vi "Benchmarking Sets.vi"() -> ()   [LabVIEW 2019]
uses:
  60997348-983d-410f-b173-2636c18fe73e.vi
  dff44dff-3936-4863-b921-07dd1a0d616c.vi
  04c840ee-3486-441b-89c1-6d55a373077b.vi
  1b5ecc8c-3254-42fc-b27c-bc730ca8b5e0.vi
  041710f1-907d-468f-a1fd-b8ae1aa895de.vi
panel:
  out "Array Intersection Count":i32
  out "Array Sym Diff Count":i32
  out "Array Union Count":i32
  out "Array Diff Count":i32
  out "Set Intersection Complete":bool=TRUE
  out "Set Intersection Started":bool=TRUE
  out "Set Symmetric Diff Complete":bool=TRUE
  out "Set Symmetric Diff Started":bool=TRUE
  out "Set Union Complete":bool=TRUE
  out "Set Union Started":bool=TRUE
  out "Set Diff Complete":bool=TRUE
  out "Set Diff Started":bool=TRUE
  out "Set Build Complete":bool=TRUE
  out "Set Build Started":bool=TRUE
  out "Array Intersection Complete":bool=TRUE
  out "Array Intersection Started":bool=TRUE
  out "Array Symmetric Diff Complete":bool=TRUE
  out "Array Symmetric Diff Started":bool=TRUE
  out "Array Union Complete":bool=TRUE
  out "Array Union Started":bool=TRUE
  out "Array Diff Complete":bool=TRUE
  out "Array Diff Started":bool=TRUE
  out "Build Arrays Complete":bool=TRUE
  out "Build Arrays Started":bool=TRUE
  out "Current iteration size":i32
  out "Outer Count":i32
  out "Inner Count":i32
  out "intersection":set{string}(c389)
  out "Set symmetric difference":set{string}(c389)
  out "Set union":set{string}(c389)
  out "Set difference":set{string}(c389)
  out "Array Intersection":string[](array[string])
  out "Array Symmetric Diff":string[](array[string])
  out "Array Union":string[](array[string])
  out "Array Diff":string[](array[string])
  out "Table operations":cluster{"Entry Count":i32[], dbl[]}[](graph)
  out "Build data sets":cluster{"Entry Count":i32[], dbl[]}[](graph)
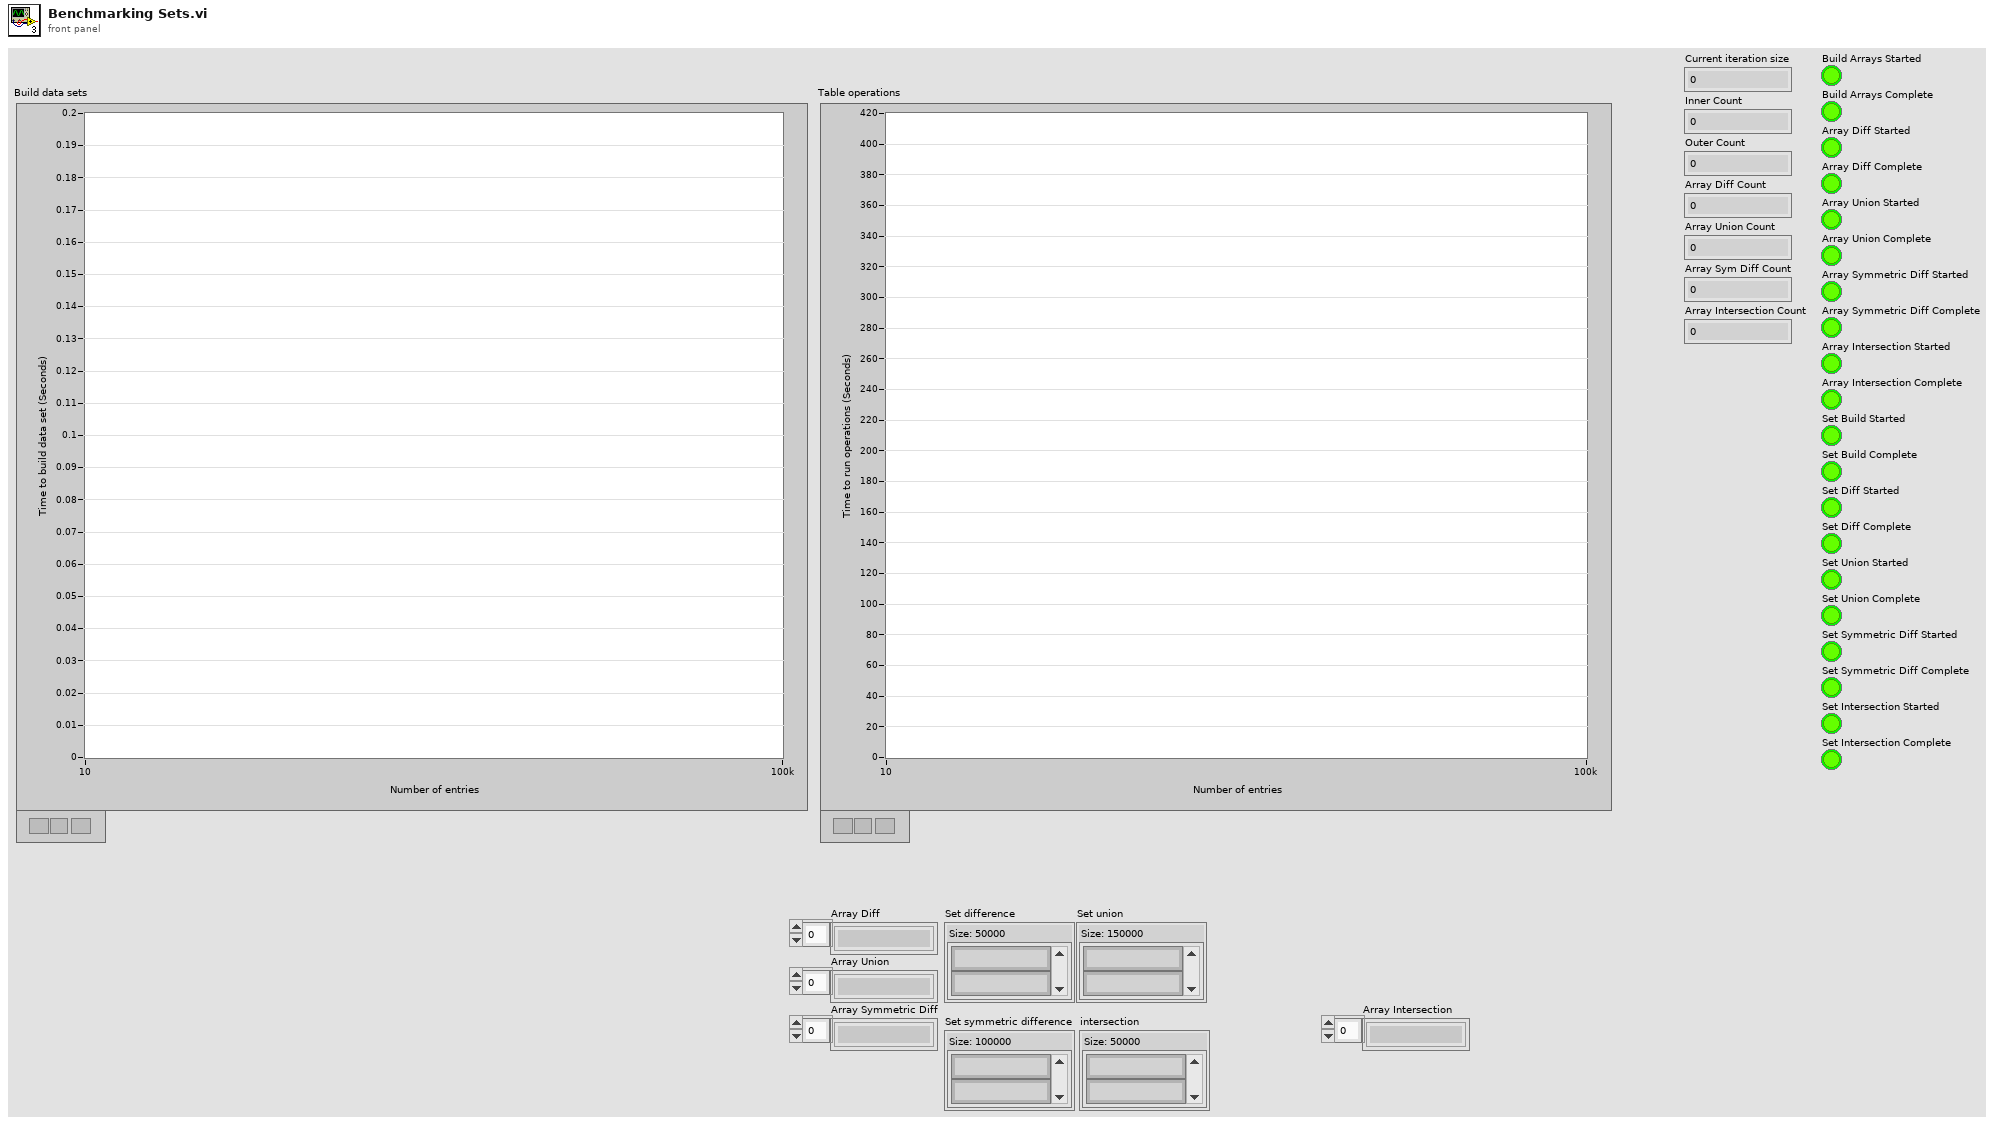
[diagram p1: front panel]
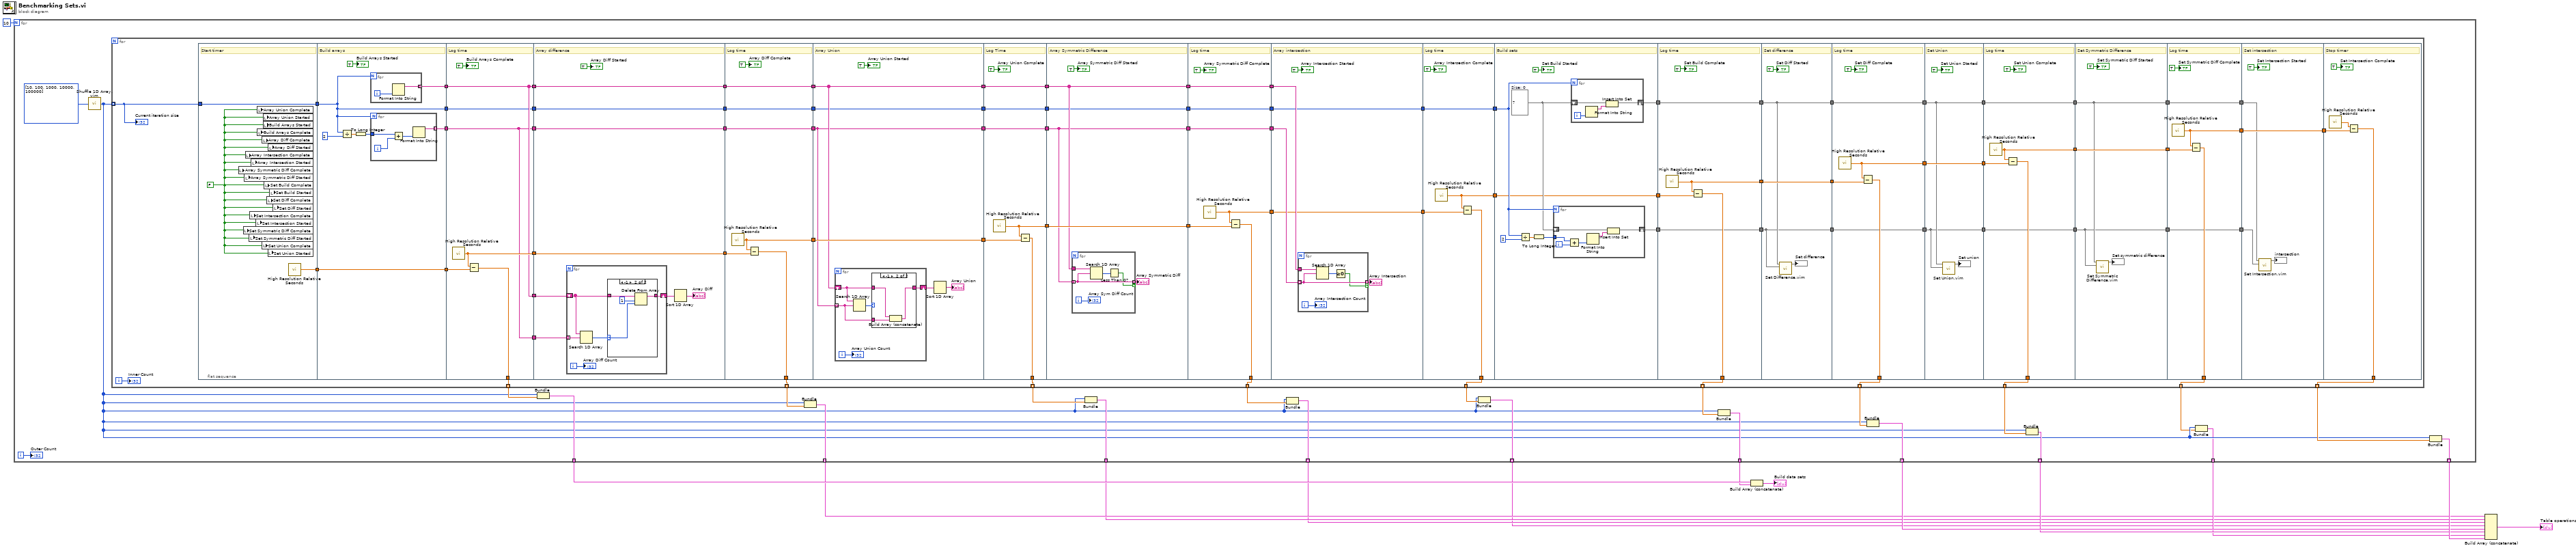
[diagram p0: block diagram]
diagram:
  n1 = for {
    N: 10 -> [_]
    tunnel: [w33] -> w12 mode=indexing
    tunnel: [w32] -> w4 mode=indexing
    tunnel: [w30] -> w11 mode=indexing
    tunnel: [w28] -> w7 mode=indexing
    tunnel: [w25] -> w6 mode=indexing
    tunnel: [w24] -> w9 mode=indexing
    tunnel: [w22] -> w3 mode=indexing
    tunnel: [w20] -> w2 mode=indexing
    tunnel: [w18] -> w1 mode=indexing
    tunnel: [w15] -> w5 mode=indexing
    i -> [w14]
    n2 = call "Shuffle 1D Array.vim"("array"=i32[] [10, 100, 1000, 10000, 100000] ("Entry Count")) -> ("shuffled array"=w17:i32[])  [unwired: 4 in]
    n3 = for {
      tunnel: [w104] -> w35 mode=indexing
      tunnel: [w103] -> w34 mode=indexing
      tunnel: [w102] -> w31 mode=indexing
      tunnel: [w101] -> w29 mode=indexing
      tunnel: [w100] -> w27 mode=indexing
      tunnel: [w99] -> w26 mode=indexing
      tunnel: w17 -> [w97] mode=indexing
      tunnel: [w84] -> w23 mode=indexing
      tunnel: [w77] -> w21 mode=indexing
      tunnel: [w70] -> w19 mode=indexing
      tunnel: [w44] -> w16 mode=indexing
      i -> [w37]
      n4 = flat-sequence {
        tunnel: [w116] -> w113
        tunnel: [w115] -> w98
        tunnel: w97 -> [w115]
        tunnel: w113 -> [w124]
        tunnel: [w124] -> w112
        tunnel: w98 -> [w118]
        tunnel: [w123] -> w95
        tunnel: [w119] -> w93
        tunnel: [w118] -> w60
        tunnel: w112 -> [w137]
        tunnel: [w136] -> w111
        tunnel: [w135] -> w104
        tunnel: [w134] -> w96
        tunnel: w95 -> [w134]
        tunnel: [w133] -> w94
        tunnel: w93 -> [w133]
        tunnel: [w134] -> w91
        tunnel: [w133] -> w86
        tunnel: [w132] -> w61
        tunnel: w60 -> [w132]
        tunnel: w111 -> [w146]
        tunnel: [w146] -> w110
        tunnel: w96 -> [w144]
        tunnel: w94 -> [w145]
        tunnel: w91 -> [w142]
        tunnel: [w142] -> w90
        tunnel: [w141] -> w87
        tunnel: w86 -> [w141]
        tunnel: [w139] -> w62
        tunnel: w61 -> [w139]
        tunnel: w110 -> [w163]
        tunnel: [w162] -> w92
        tunnel: [w161] -> w103
        tunnel: w90 -> [w160]
        tunnel: [w160] -> w89
        tunnel: [w159] -> w88
        tunnel: w87 -> [w159]
        tunnel: [w158] -> w63
        tunnel: w62 -> [w158]
        tunnel: w92 -> [w170]
        tunnel: [w170] -> w85
        tunnel: w89 -> [w167]
        tunnel: w88 -> [w166]
        tunnel: [w167] -> w82
        tunnel: [w166] -> w80
        tunnel: [w165] -> w64
        tunnel: w63 -> [w165]
        tunnel: w85 -> [w186]
        tunnel: [w185] -> w84
        tunnel: [w184] -> w83
        tunnel: w82 -> [w184]
        tunnel: [w183] -> w81
        tunnel: w80 -> [w183]
        tunnel: [w182] -> w78
        tunnel: [w181] -> w65
        tunnel: w64 -> [w181]
        tunnel: w83 -> [w190]
        tunnel: w81 -> [w189]
        tunnel: [w191] -> w79
        tunnel: w78 -> [w191]
        tunnel: [w190] -> w76
        tunnel: [w189] -> w73
        tunnel: [w188] -> w66
        tunnel: w65 -> [w188]
        tunnel: w79 -> [w204]
        tunnel: [w203] -> w77
        tunnel: w76 -> [w202]
        tunnel: [w202] -> w75
        tunnel: [w201] -> w74
        tunnel: w73 -> [w201]
        tunnel: [w200] -> w71
        tunnel: [w199] -> w67
        tunnel: w66 -> [w199]
        tunnel: w75 -> [w209]
        tunnel: w74 -> [w208]
        tunnel: [w207] -> w72
        tunnel: w71 -> [w207]
        tunnel: [w206] -> w68
        tunnel: w67 -> [w206]
        tunnel: w72 -> [w220]
        tunnel: [w219] -> w70
        tunnel: [w218] -> w69
        tunnel: w68 -> [w218]
        tunnel: [w217] -> w58
        tunnel: w69 -> [w227]
        tunnel: [w224] -> w59
        tunnel: w58 -> [w224]
        tunnel: [w223] -> w57
        tunnel: [w222] -> w54
        tunnel: [w245] -> w109
        tunnel: [w244] -> w102
        tunnel: w59 -> [w243]
        tunnel: w57 -> [w242]
        tunnel: [w242] -> w56
        tunnel: [w241] -> w55
        tunnel: w54 -> [w241]
        tunnel: w109 -> [w250]
        tunnel: [w250] -> w108
        tunnel: w56 -> [w248]
        tunnel: w55 -> [w247]
        tunnel: [w248] -> w53
        tunnel: [w247] -> w50
        tunnel: w108 -> [w256]
        tunnel: [w255] -> w107
        tunnel: [w254] -> w101
        tunnel: w53 -> [w253]
        tunnel: [w253] -> w52
        tunnel: [w252] -> w51
        tunnel: w50 -> [w252]
        tunnel: w107 -> [w261]
        tunnel: [w261] -> w106
        tunnel: w52 -> [w259]
        tunnel: w51 -> [w258]
        tunnel: [w259] -> w49
        tunnel: [w258] -> w47
        tunnel: w106 -> [w267]
        tunnel: [w266] -> w105
        tunnel: [w265] -> w100
        tunnel: w49 -> [w264]
        tunnel: [w264] -> w48
        tunnel: w47 -> [w263]
        tunnel: [w263] -> w46
        tunnel: w105 -> [w271]
        tunnel: w48 -> [w270]
        tunnel: w46 -> [w269]
        tunnel: [w271] -> w45
        tunnel: [w270] -> w41
        tunnel: [w269] -> w38
        tunnel: w45 -> [w278]
        tunnel: [w277] -> w44
        tunnel: [w276] -> w42
        tunnel: w41 -> [w275]
        tunnel: [w275] -> w40
        tunnel: [w274] -> w39
        tunnel: w38 -> [w274]
        tunnel: [w283] -> w43
        tunnel: w42 -> [w283]
        tunnel: w40 -> [w282]
        tunnel: w39 -> [w281]
        tunnel: [w286] -> w99
        tunnel: w43 -> [w285]
        frame #0 {
          w114 = FALSE ("Build Arrays Started")
          # "Start timer"
          n5 = local write "Array Symmetric Diff Complete"(w114) -> ()
          n6 = local write "Set Symmetric Diff Complete"(w114) -> ()
          n7 = local write "Array Symmetric Diff Started"(w114) -> ()
          n8 = local write "Array Intersection Complete"(w114) -> ()
          n9 = local write "Set Symmetric Diff Started"(w114) -> ()
          n10 = local write "Set Intersection Complete"(w114) -> ()
          n11 = local write "Array Intersection Started"(w114) -> ()
          n12 = local write "Set Intersection Started"(w114) -> ()
          n13 = local write "Array Union Complete"(w114) -> ()
          n14 = local write "Build Arrays Complete"(w114) -> ()
          n15 = local write "Set Union Complete"(w114) -> ()
          n16 = local write "Array Diff Complete"(w114) -> ()
          n17 = local write "Array Union Started"(w114) -> ()
          n18 = local write "Build Arrays Started"(w114) -> ()
          n19 = local write "Set Build Complete"(w114) -> ()
          n20 = local write "Set Diff Complete"(w114) -> ()
          n21 = local write "Set Union Started"(w114) -> ()
          n22 = local write "Array Diff Started"(w114) -> ()
          n23 = local write "Set Build Started"(w114) -> ()
          n24 = local write "Set Diff Started"(w114) -> ()
          n25 = call <vilib>:"High Resolution Relative Seconds.vi"() -> ("relative seconds"=w116:dbl)
        }
        frame #1 {
          # "Build arrays"
          n26 = Divide(x=w118, y=2) -> (x/y=w121:dbl)
          n27 = To Long Integer(number=w121) -> (32bit integer=w120:i32)
          n28 = for {
            N: w118 -> [_]
            tunnel: [w129] -> w123 mode=indexing
            i -> [w130]
            n29 = Format Into String(w130) -> (resulting string=w129:string)  [unwired: 3 in, 1 out]
          }
          n30 = for {
            N: w118 -> [_]
            tunnel: [w126] -> w119 mode=indexing
            tunnel: w120 -> [w127]
            i -> [w128]
            n31 = Add(x=w127, y=w128) -> (x+y=w125:i32)
            n32 = Format Into String(w125) -> (resulting string=w126:string)  [unwired: 3 in, 1 out]
          }
          "Build Arrays Started" <- TRUE
        }
        frame #2 {
          # "Log time"
          n33 = call <vilib>:"High Resolution Relative Seconds.vi"() -> ("relative seconds"=w136:dbl)
          n34 = Subtract(x=w136, y=w137) -> (x-y=w135:dbl)
          "Build Arrays Complete" <- TRUE
        }
        frame #3 {
          # "Array difference"
          n35 = for {
            tunnel: w145 -> [w151] mode=indexing
            shift-right: [w148] -> w143
            shift-left: w144 -> [w149]
            i -> [w147]
            n36 = Search 1D Array(1D array=w149, element=w151) -> (index of element=w150:i32)  [unwired: 1 in]
            n37 = case shown="-1" w150 {
              selector: w150 -> [_ w153]
              tunnel: w149 -> [w152 w156]
              tunnel: [w152 w155] -> w148
              frame Default {
              }
              frame -1 {
                n38 = Delete From Array(array=w156, length=1, index=w153) -> (array with subset deleted=w155:string[])  [unwired: 1 out]
              }
            }
            "Array Diff Count" <- w147
          }
          n39 = Sort 1D Array(array=w143) -> (sorted array=→"Array Diff":string[])
          "Array Diff Started" <- TRUE
        }
        frame #4 {
          # "Log time"
          n40 = call <vilib>:"High Resolution Relative Seconds.vi"() -> ("relative seconds"=w162:dbl)
          n41 = Subtract(x=w162, y=w163) -> (x-y=w161:dbl)
          "Array Diff Complete" <- TRUE
        }
        frame #5 {
          # "Array Union"
          n42 = for {
            shift-right: [w173] -> w169
            shift-left: w167 -> [w174]
            tunnel: w166 -> [w172] mode=indexing
            i -> [w171]
            n43 = Search 1D Array(1D array=w174, element=w172) -> (index of element=w175:i32)  [unwired: 1 in]
            n44 = case shown="-1" w175 {
              tunnel: w174 -> [w176 w179]
              tunnel: [w176 w178] -> w173
              tunnel: w172 -> [_ w177]
              frame Default {
              }
              frame -1 {
                n45 = Build Array (concatenate)(w179, w177) -> (w178:string[])
              }
            }
            "Array Union Count" <- w171
          }
          n46 = Sort 1D Array(array=w169) -> (sorted array=→"Array Union":string[])
          "Array Union Started" <- TRUE
        }
        frame #6 {
          # "Log Time"
          n47 = call <vilib>:"High Resolution Relative Seconds.vi"() -> ("relative seconds"=w182:dbl)
          n48 = Subtract(x=w182, y=w186) -> (x-y=w185:dbl)
          "Array Union Complete" <- TRUE
        }
        frame #7 {
          # "Array Symmetric Difference"
          n49 = for {
            tunnel: w190 -> [w197]
            tunnel: w189 -> [w195] mode=indexing
            tunnel: [w195] -> w192 mode=indexing if=w194
            i -> [w193]
            n50 = Search 1D Array(1D array=w197, element=w195) -> (index of element=w196:i32)  [unwired: 1 in]
            n51 = Less Than 0?(x=w196) -> (x < 0?=w194:bool)
            "Array Sym Diff Count" <- w193
          }
          "Array Symmetric Diff" <- w192
          "Array Symmetric Diff Started" <- TRUE
        }
        frame #8 {
          # "Log time"
          n52 = call <vilib>:"High Resolution Relative Seconds.vi"() -> ("relative seconds"=w200:dbl)
          n53 = Subtract(x=w200, y=w204) -> (x-y=w203:dbl)
          "Array Symmetric Diff Complete" <- TRUE
        }
        frame #9 {
          # "Array intersection"
          n54 = for {
            tunnel: w209 -> [w215]
            tunnel: w208 -> [w213] mode=indexing
            tunnel: [w213] -> w210 mode=indexing if=w212
            i -> [w211]
            n55 = Search 1D Array(1D array=w215, element=w213) -> (index of element=w214:i32)  [unwired: 1 in]
            n56 = Greater Or Equal To 0?(x=w214) -> (x >= 0?=w212:bool)
            "Array Intersection Count" <- w211
          }
          "Array Intersection" <- w210
          "Array Intersection Started" <- TRUE
        }
        frame #10 {
          # "Log time"
          n57 = call <vilib>:"High Resolution Relative Seconds.vi"() -> ("relative seconds"=w217:dbl)
          n58 = Subtract(x=w217, y=w220) -> (x-y=w219:dbl)
          "Array Intersection Complete" <- TRUE
        }
        frame #11 {
          w225 = set{string} {}  # Size: 0
          # "Build sets"
          n59 = Divide(x=w227, y=2) -> (x/y=w228:dbl)
          n60 = To Long Integer(number=w228) -> (32bit integer=w226:i32)
          n61 = for {
            N: w227 -> [_]
            shift-right: [w232] -> w222
            shift-left: w225 -> [w235]
            tunnel: w226 -> [w230]
            i -> [w234]
            n62 = Add(x=w230, y=w234) -> (x+y=w231:i32)
            n63 = Format Into String(w231) -> (resulting string=w233:string)  [unwired: 3 in, 1 out]
            n64 = Insert Into Set(10:w233, 11:w235) -> (3:w232:set{string})  [unwired: 1 out]
          }
          n65 = for {
            N: w227 -> [_]
            shift-right: [w236] -> w223
            shift-left: w225 -> [w239]
            i -> [w238]
            n66 = Format Into String(w238) -> (resulting string=w237:string)  [unwired: 3 in, 1 out]
            n67 = Insert Into Set(10:w237, 11:w239) -> (3:w236:set{string})  [unwired: 1 out]
          }
          "Set Build Started" <- TRUE
        }
        frame #12 {
          # "Log time"
          n68 = call <vilib>:"High Resolution Relative Seconds.vi"() -> ("relative seconds"=w245:dbl)
          n69 = Subtract(x=w245, y=w243) -> (x-y=w244:dbl)
          "Set Build Complete" <- TRUE
        }
        frame #13 {
          # "Set difference"
          n70 = call "Set Difference.vim"("set 2"=w247, "set 1"=w248) -> ("difference"=→"Set difference":set{string})  [unwired: 9 in]
          "Set Diff Started" <- TRUE
        }
        frame #14 {
          # "Log time"
          n71 = call <vilib>:"High Resolution Relative Seconds.vi"() -> ("relative seconds"=w255:dbl)
          n72 = Subtract(x=w255, y=w256) -> (x-y=w254:dbl)
          "Set Diff Complete" <- TRUE
        }
        frame #15 {
          # "Set Union"
          n73 = call "Set Union.vim"("set 2"=w258, "set 1"=w259) -> ("union"=→"Set union":set{string})  [unwired: 9 in]
          "Set Union Started" <- TRUE
        }
        frame #16 {
          # "Log time"
          n74 = call <vilib>:"High Resolution Relative Seconds.vi"() -> ("relative seconds"=w266:dbl)
          n75 = Subtract(x=w266, y=w267) -> (x-y=w265:dbl)
          "Set Union Complete" <- TRUE
        }
        frame #17 {
          # "Set Symmetric Difference"
          n76 = call "Set Symmetric Difference.vim"("set 2"=w269, "set 1"=w270) -> ("symmetric difference"=→"Set symmetric difference":set{string})  [unwired: 9 in]
          "Set Symmetric Diff Started" <- TRUE
        }
        frame #18 {
          # "Log time"
          n77 = call <vilib>:"High Resolution Relative Seconds.vi"() -> ("relative seconds"=w276:dbl)
          n78 = Subtract(x=w276, y=w278) -> (x-y=w277:dbl)
          "Set Symmetric Diff Complete" <- TRUE
        }
        frame #19 {
          # "Set intersection"
          n79 = call "Set Intersection.vim"("set 2"=w281, "set 1"=w282) -> ("intersection"=→"intersection":set{string})  [unwired: 9 in]
          "Set Intersection Started" <- TRUE
        }
        frame #20 {
          # "Stop timer"
          n80 = call <vilib>:"High Resolution Relative Seconds.vi"() -> ("relative seconds"=w287:dbl)
          n81 = Subtract(x=w287, y=w285) -> (x-y=w286:dbl)
          "Set Intersection Complete" <- TRUE
        }
      }
      "Inner Count" <- w37
      "Current iteration size" <- w97
    }
    n82 = Bundle("shuffled array"=w17, w35) -> (w33:cluster{"shuffled array":i32[], dbl[]})  [unwired: 1 in]
    n83 = Bundle("shuffled array"=w17, w34) -> (w32:cluster{"shuffled array":i32[], dbl[]})  [unwired: 1 in]
    n84 = Bundle("shuffled array"=w17, w23) -> (w22:cluster{"shuffled array":i32[], dbl[]})  [unwired: 1 in]
    n85 = Bundle("shuffled array"=w17, w21) -> (w20:cluster{"shuffled array":i32[], dbl[]})  [unwired: 1 in]
    n86 = Bundle("shuffled array"=w17, w19) -> (w18:cluster{"shuffled array":i32[], dbl[]})  [unwired: 1 in]
    n87 = Bundle("shuffled array"=w17, w31) -> (w30:cluster{"shuffled array":i32[], dbl[]})  [unwired: 1 in]
    n88 = Bundle("shuffled array"=w17, w29) -> (w28:cluster{"shuffled array":i32[], dbl[]})  [unwired: 1 in]
    n89 = Bundle("shuffled array"=w17, w27) -> (w25:cluster{"shuffled array":i32[], dbl[]})  [unwired: 1 in]
    n90 = Bundle("shuffled array"=w17, w16) -> (w15:cluster{"shuffled array":i32[], dbl[]})  [unwired: 1 in]
    n91 = Bundle("shuffled array"=w17, w26) -> (w24:cluster{"shuffled array":i32[], dbl[]})  [unwired: 1 in]
    "Outer Count" <- w14
  }
  n92 = Build Array (concatenate)(w12, w11) -> (→"Build data sets":cluster{"shuffled array":i32[], dbl[]}[])
  n93 = Build Array (concatenate)(w4, w3, w2, w1, w7, w6, w5, w9) -> (→"Table operations":cluster{"shuffled array":i32[], dbl[]}[])
